vi "Destroy Test Suite.vi"(8 "error in (no error)":errorcluster, 11 "Test Suite in":refnum<class "Test Suite.lvclass">) -> (0 "error out":errorcluster)   [LabVIEW 2009, in "Caraya.lvlib" / "Test Suite.lvclass"]
doc: "Destroys a test suite.\n\n--\nCopyright © 2015 JKI All rights reserved.\n\nAuthor: Tomi Maila <tomi.maila@jki.net>\n\nThis library is provided \"AS IS\" ,WITHOUT WARRANTIES OR\nCONDITIONS OF ANY KIND, either express or implied.\n\nJKI -- jki.net"
uses:
  Test Suite.lvclass
  Test Suite.lvclass/Test Suite.ctl
  Test Manager/Test Manager.lvclass
panel:
  # "Copyright © 2015 JKI All rights reserved.\n\nAuthor: Tomi Maila <tomi.maila@jki.net>\n\nThis library is provided \"AS IS\" ,WITHOUT WARRANTIES OR\nCONDITIONS OF ANY KIND, either express or implied.\n\nJKI -- jki.net"
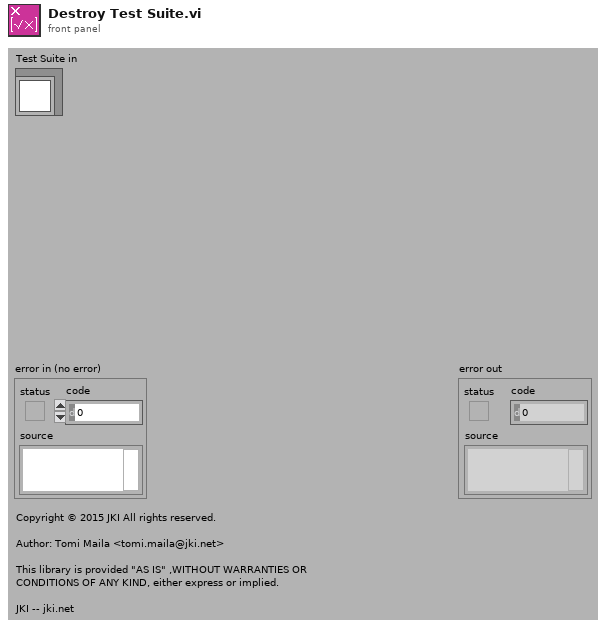
[diagram p1: front panel]
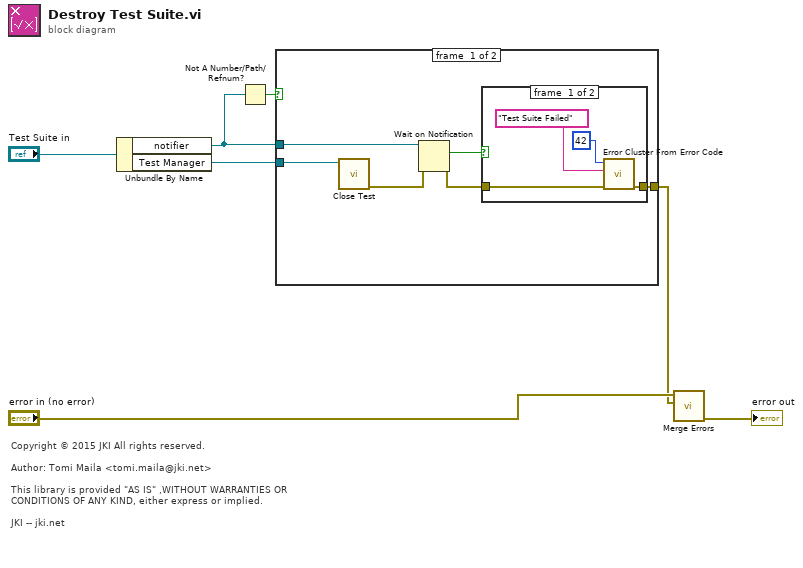
[diagram p0: block diagram]
diagram:
  # "Copyright © 2015 JKI All rights reserved.\n\nAuthor: Tomi Maila <tomi.maila@jki.net>\n\nThis library is provided \"AS IS\" ,WITHOUT WARRANTIES OR\nCONDITIONS OF ANY KIND, either express or implied.\n\nJKI -- jki.net"
  n1 = Unbundle By Name("Test Suite in") -> ("notifier"=w1:refnum<notifier>, "Test Manager"=w6:refnum<class "Test Manager.lvclass">)
  n2 = Not A Number/Path/Refnum?(number/path/refnum=w1) -> (NaN/Path/Refnum?=w2:bool)
  n3 = case shown="False" w2 {
    tunnel: w6 -> [w13 _]
    tunnel: [w11 _] -> w3
    tunnel: w1 -> [w8 _]
    frame #0 {
      n4 = call-dynamic "Close Test.vi"("Test Manager in"=w13) -> ("error out"=w12:errorcluster)  [unwired: 9 in, 1 out]
      n5 = Wait on Notification(notifier=w8, error in (no error)=w12) -> (notification=w9:bool, error out=w10:errorcluster)  [unwired: 2 in, 2 out]
      n6 = case shown="False" w9 {
        tunnel: [w17 w18] -> w11
        tunnel: w10 -> [w16 w18]
        frame #0 {
          n7 = call <vilib>:"Error Cluster From Error Code.vi"("error in (no error)"=w16, "error message (\"\")"="Test Suite Failed" ("error message (\"\")"), "error code (0)"=42) -> ("error out"=w17:errorcluster)  [unwired: 6 in]
        }
        frame #1 {
        }
      }
    }
    frame #1 {
    }
  }
  n8 = call <vilib>:"Merge Errors.vi"("error in 2 (no error)"=w3, "error in 1 (no error)"="error in (no error)") -> ("error out"=→"error out":errorcluster)  [unwired: 5 in]
